vi "Instrument.Lockin.getAO.vi"(8 "error in (no error)":errorcluster, 11 "Instrument.Lockin in":refnum<class "Instrument.Lockin.lvclass">) -> (0 "error out":errorcluster, 3 "Instrument.Lockin out":refnum<class "Instrument.Lockin.lvclass">)   [LabVIEW 2019, in "Instrument.Lockin.lvclass"]
uses:
  Instrument.Lockin.lvclass
  Typedefs/PublicEvents--Instrument.Lockin.getAO.ctl
panel:
  in  "getAO":T1
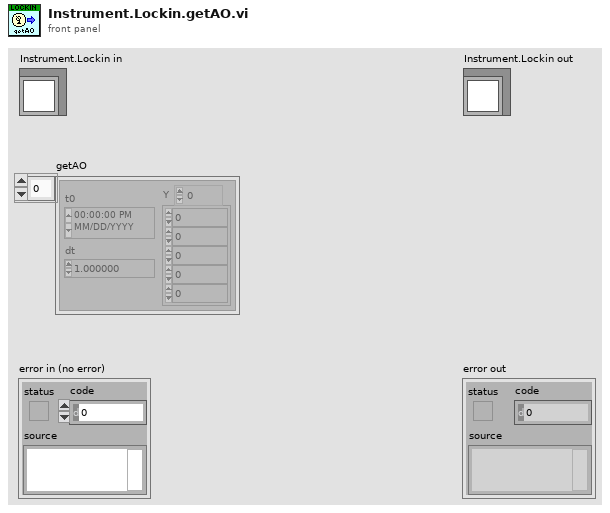
[diagram p1: front panel]
types:
  T1 = typedef "Instrument.Lockin.lvclass/PublicEvents--Instrument.Lockin.getAO.ctl" = waveform(dbl)[]
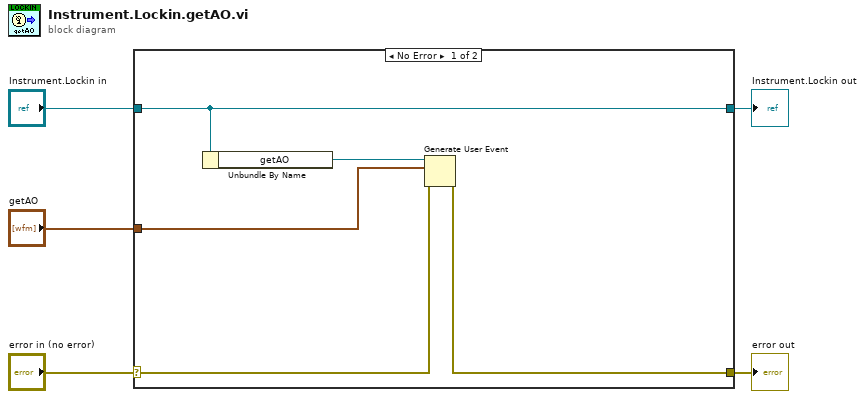
[diagram p0: block diagram]
diagram:
  n1 = case shown="No Error" "error in (no error)" {
    selector: "error in (no error)" -> [w7 w12]
    tunnel: [w6 w12] -> w4
    tunnel: [w10 w11] -> w2
    tunnel: "Instrument.Lockin in" -> [w10 w11]
    tunnel: "getAO" -> [w8 _]
    frame No Error {
      n2 = Unbundle By Name(w10) -> ("getAO"=w9:refnum<user-event>)
      n3 = Generate User Event(user event=w9, event data cluster=w8, error in=w7) -> (error out=w6:errorcluster)  [unwired: 1 in, 1 out]
    }
    frame Error {
    }
  }
  "error out" <- w4
  "Instrument.Lockin out" <- w2
